vi "Fetch Voltages.vi"(8 "error in":errorcluster, 11 "OWON SDS1022 in":refnum<class "OWON SDS1022.lvclass">) -> (0 "error out":errorcluster, 3 "OWON SDS1022 out":refnum<class "OWON SDS1022.lvclass">)   [LabVIEW 2023, in "OWON SDS1022.lvlib" / "OWON SDS1022.lvclass"]
uses:
  OWON SDS1022.lvclass
  E:/git/HAL/Scope Base/Scope Base.lvclass
  HAL/Scope Base/Scope Base.lvclass/Scope Base.ctl
  <vilib>/Analysis/baseanly.llb/Mean (DBL).vi
  HAL/Scope Base/Scope Base.lvclass
  <vilib>/Analysis/NI_AALBase.lvlib
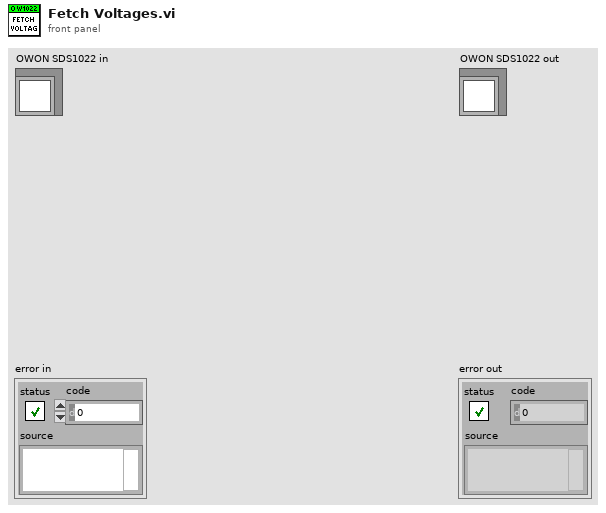
[diagram p1: front panel]
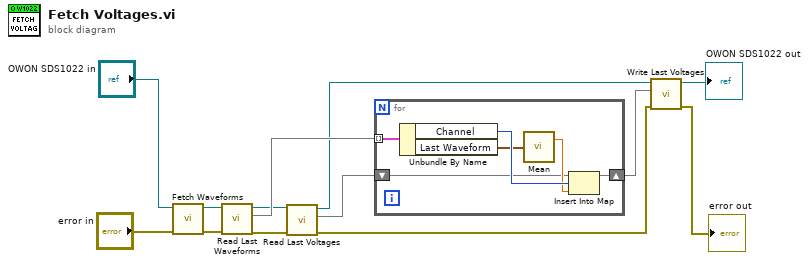
[diagram p0: block diagram]
diagram:
  n1 = call-dynamic "Fetch Waveforms.vi"("error in (no error)"="error in", "OWON SDS1022 in"="OWON SDS1022 in") -> ("error out"=w12:errorcluster, "OWON SDS1022 out"=w10:refnum<class "OWON SDS1022.lvclass">)  [unwired: 8 in]
  n2 = call "Read Last Waveforms.vi"("error in (no error)"=w12, "Scope Base in"=w10) -> ("error out"=w8:errorcluster, "Last Waveforms"=w9:map{u8, waveform(dbl)}, "Scope Base out"=w7:refnum<class "OWON SDS1022.lvclass">)  [unwired: 7 in]
  n3 = call "Read Last Voltages.vi"("error in (no error)"=w8, "Scope Base in"=w7) -> ("error out"=w5:errorcluster, "Last Voltage"=w6:map{u8, dbl}, "Scope Base out"=w3:refnum<class "OWON SDS1022.lvclass">)  [unwired: 7 in]
  n4 = for {
    tunnel: w9 -> [w19] mode=indexing
    shift-right: [w14] -> w1
    shift-left: w6 -> [w15]
    n5 = Unbundle By Name(w19) -> ("Channel"=w18:u8, "Last Waveform"=w17:waveform(dbl))
    n6 = call-poly <vilib>:"Mean.vi"("X"=w17) -> ("mean"=w16:dbl)  [unwired: 1 out]
    n7 = Insert Into Map(map in=w15, key=w18, value=w16) -> (map out=w14:map{u8, dbl})  [unwired: 2 out]
  }
  n8 = call "Write Last Voltages.vi"("error in (no error)"=w5, "Last Voltage"=w1, "Scope Base in"=w3) -> ("error out"=→"error out":errorcluster, "Scope Base out"=→"OWON SDS1022 out":refnum<class "OWON SDS1022.lvclass">)  [unwired: 7 in]
